vi "날짜_그래프_시험.vi"() -> ()   [LabVIEW 2024]
panel:
  out "추가된 배열":dbl[](array[numeric])
  out "웨이브폼 차트":waveform(dbl)(graph)
  out "웨이브폼 그래프":waveform(dbl)(graph)
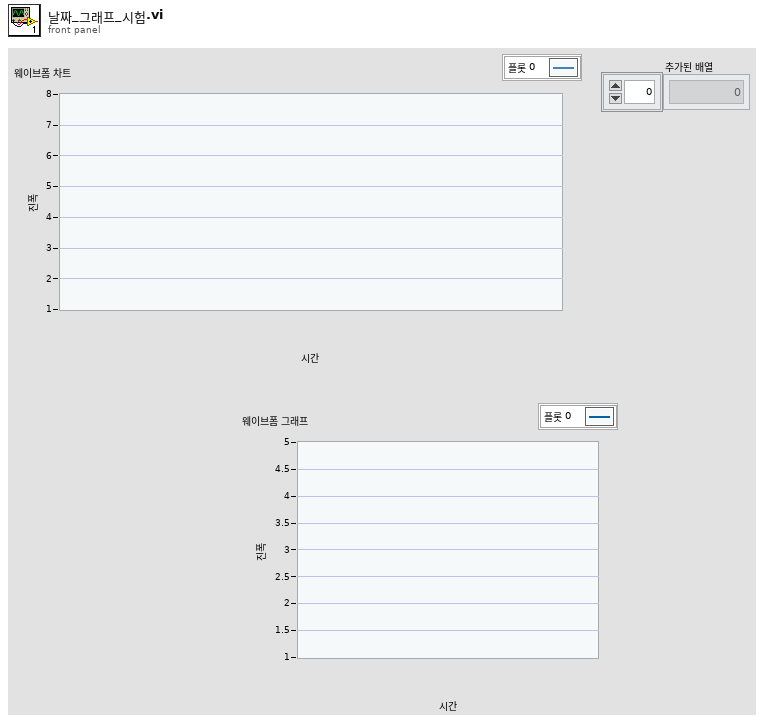
[diagram p1: front panel]
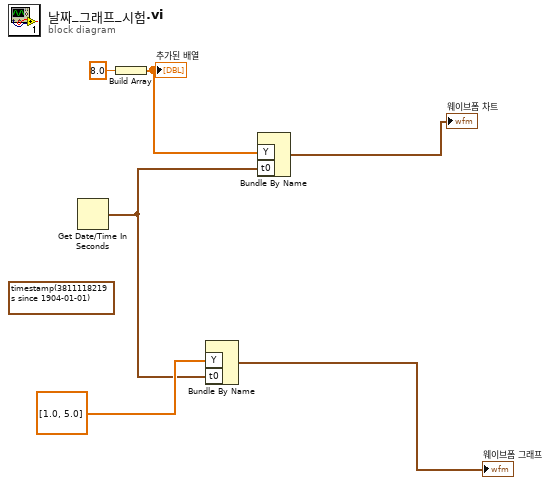
[diagram p0: block diagram]
diagram:
  (unwired) timestamp(3811118219 s since 1904-01-01) ("t0")
  n1 = Get Date/Time In Seconds() -> (seconds since 1Jan1904=w4:timestamp)
  n2 = Build Array(8.0 ("원소")) -> (w1:dbl[])
  "추가된 배열" <- w1
  n3 = Bundle By Name("Y"=dbl[] [1.0, 5.0], "t0"=w4) -> (→"웨이브폼 그래프":waveform(dbl))  [unwired: 1 in]
  n4 = Bundle By Name("Y"=w1, "t0"=w4) -> (→"웨이브폼 차트":waveform(dbl))  [unwired: 1 in]
